vi "NetworkServerDiscoverywithPassword.vi"() -> ()   [LabVIEW 2012, in "Phidget Common.lvlib"]
uses:
  <instrlib>/Phidgets/Phidget Common/Phidget Common.lvlib
  <instrlib>/Phidgets/Phidget Accelerometer/Public/AccelerometerStart.vi
  <instrlib>/Phidgets/Phidget Accelerometer/Public/AccelerometerClose.vi
  <instrlib>/Phidgets/Phidget Accelerometer/Phidget Accelerometer.lvlib
panel:
  out "Acceleration":dbl[](array[numeric])
  out "error out":errorcluster
  in  "Device Info":T1={"Serial Number"=-1, "Channel"=0, "Port"=0}
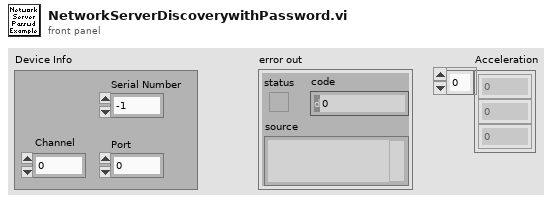
[diagram p1: front panel]
types:
  T1 = cluster{"Serial Number":i32, "Channel":i32, "Port":i32}
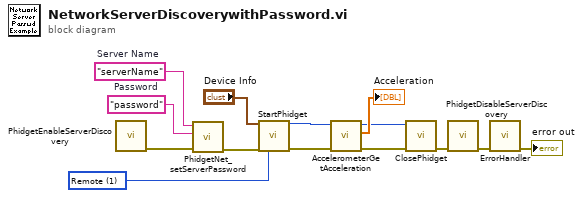
[diagram p0: block diagram]
diagram:
  w1 = "password"  # Password
  w2 = "serverName"  # Server Name
  w14 = u16 1 items=["No Preference", "Remote", "Local"] ("Connection")
  n1 = call <instrlib>:"PhidgetEnableServerDiscovery.vi"() -> ("error out"=w4:errorcluster)  [unwired: 11 in]
  n2 = call <instrlib>:"PhidgetNet_setServerPassword.vi"("error in"=w4, "Password"=w1, "Server Name"=w2) -> ("error out"=w3:errorcluster)  [unwired: 8 in]
  n3 = call-poly <instrlib>:"StartPhidget.vi"("Device Info"="Device Info", "error in (no error)"=w3, "Connection"=w14) -> ("Phidget ID"=w8:u64, "error out"=w7:errorcluster)  [unwired: 9 in, 2 out]
  n4 = call <instrlib>:"AccelerometerGetAcceleration.vi"("error in (no error)"=w7, "Device In"=w8) -> ("error out"=w6:errorcluster, "Acceleration"=→"Acceleration":dbl[], "Device Out"=w5:u64)  [unwired: 6 in]
  n5 = call-poly <instrlib>:"ClosePhidget.vi"("error in"=w6, "Device In"=w5) -> ("error out"=w12:errorcluster)  [unwired: 9 in]
  n6 = call <instrlib>:"PhidgetDisableServerDiscovery.vi"("error in"=w12) -> ("error out"=w11:errorcluster)  [unwired: 10 in]
  n7 = call <instrlib>:"ErrorHandler.vi"("error in"=w11) -> ("error out"=→"error out":errorcluster)  [unwired: 9 in, 1 out]
